vi "FIR Windowed (Uniform) Filter Coefficients.vi"(0 "sampling freq: fs":dbl=1.0 format="%0.2f", 1 "filter type":T1, 2 "high cutoff freq: fh":dbl=0.45 format="%0.2f", 3 "low cutoff freq: fl":dbl=0.125 format="%0.2f", 4 "taps":i32=25) -> (5 "FIR Coefficients":dbl[](array[numeric]) format="%0.2f", 6 "error":i32)   [LabVIEW 2020, in "NI_AALBase.lvlib"]
doc: "Generates the set of coefficients to implement an FIR filter."
uses:
  <vilib>/Analysis/NI_AALBase.lvlib
  <vilib>/Analysis/3filter.llb/Filter Passband Type.ctl
  <resource>/lvanlys.dll
panel:
  # "FIR Windowed (Uniform) Filter Coefficients"
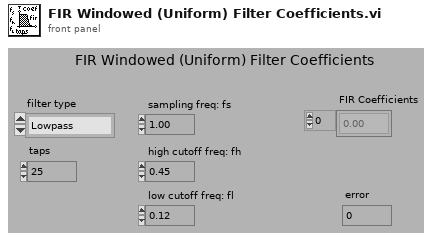
[diagram p1: front panel]
types:
  T1 = typedef "NI_AALBase.lvlib/Filter Passband Type.ctl" = enum32{"Lowpass", "Highpass", "Bandpass", "Bandstop"}
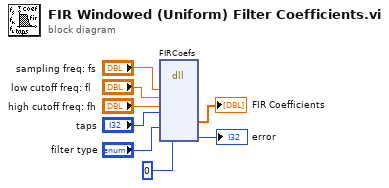
[diagram p0: block diagram]
diagram:
  n1 = dll-call lib="e:/builds/penguin/labview/branches/2020/dev/dist/resource/lvanlys.*" fn="FIRCoefs"("sampling freq: fs"="sampling freq: fs", "low cutoff freq: fl"="low cutoff freq: fl", "high cutoff freq: fh"="high cutoff freq: fh", "taps"="taps", "filter type"="filter type", 0) -> ("FIR Coefficients"=→"FIR Coefficients":dbl[], →"error":i32)  [unwired: 8 in, 4 out]
